vi "Build message.vi"(1 "Input string":string) -> (0 "Output string":string)   [LabVIEW 2021]
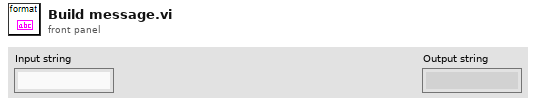
[diagram p1: front panel]
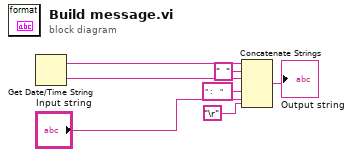
[diagram p0: block diagram]
diagram:
  n1 = Get Date/Time String() -> (date string=w7:string, time string=w5:string)  [unwired: 3 in]
  n2 = Concatenate Strings(w7, "  " ("string"), w5, " :    " ("string"), "Input string", "\r") -> (→"Output string":string)
